vi "RomiSim_Write_Sensors.vi"(10 "Diff Drive Train Sim":T8 {"m_Motor"."Jr_KgM2" format="%13.5p"; "m_Motor"."L_H" format="%13.5p"; "m_Motor"."Kt_NMPerAmp" format="%13.5p"; "m_Motor"."KvINV_RadPerSecPerVolt" format="%13.5p"; "m_Motor"."R_Ohms" format="%13.5p"; "m_Motor"."FreeSpeed_RadPerSec" format="%13.5p"; "m_Motor"."FreeCurrent_Amps" format="%13.5p"; "m_Motor"."StallCurrent_Amps" format="%13.5p"; "m_Motor"."StallTorque_NM" format="%13.5p"; "m_Motor"."nominalVoltage_Volts" format="%13.5p"}, 11 "Counts/Feet":dbl) -> (0 "Right Speed Ft/Sec":dbl, 1 "Right Encoder":T6, 2 "Left Speed Ft/Sec":dbl, 3 "Left Encoder":T6, 4 "Robot Pose":T3 {"ROTATION"."SIN" format="%13.4f"; "ROTATION"."COS" format="%13.4f"; "ROTATION"."VALUE" format="%13.4f"; "TRANSLATION"."Y" format="%14.3f"; "TRANSLATION"."X" format="%14.3f"}, 5 "Gyro Deg":dbl, 7 "Gyro":T1)   [LabVIEW 2019]
uses:
  <vilib>/Rock Robotics/WPI/ThirdParty/JAS_Junk/TrajLib/TypeDef/DIFF_DRIVE_TRAIN_SIM.ctl
  <vilib>/Rock Robotics/WPI/ThirdParty/JAS_Junk/TrajLib/TypeDef/LINEAR_SYSTEM.ctl
  <vilib>/Analysis/Matrix/Datatypes/RealMatrix.ctl
  <vilib>/Rock Robotics/WPI/ThirdParty/JAS_Junk/TrajLib/TypeDef/DCMOTOR.CTL
  <vilib>/Rock Robotics/WPI/Simulation/Protocol/Devices/Encoder/Encoder proto.ctl
  <vilib>/Rock Robotics/WPI/Simulation/Protocol/Devices/Encoder/Encoder data protoo.ctl
  <vilib>/Rock Robotics/WPI/ThirdParty/JAS_Junk/TrajLib/TypeDef/POSE2D.ctl
  <vilib>/Rock Robotics/WPI/ThirdParty/JAS_Junk/TrajLib/TypeDef/TRANSLATION2D.ctl
  <vilib>/Rock Robotics/WPI/ThirdParty/JAS_Junk/TrajLib/TypeDef/ROTATION2D.ctl
  <vilib>/Rock Robotics/WPI/Simulation/Protocol/Devices/Gyro/Gyro proto.ctl
  <vilib>/Rock Robotics/WPI/Simulation/Protocol/Devices/Gyro/Gyro Data proto.ctl
  <vilib>/Rock Robotics/WPI/Simulation/Protocol/Devices/Encoder/Encoder Update Ops.ctl
  <vilib>/Rock Robotics/SystemInterfaces/Encoder/FPGA_EncoderIdx.ctl
  <vilib>/Rock Robotics/WPI/Simulation/Protocol/Devices/Gyro/Gyro Update Ops.ctl
  <vilib>/Rock Robotics/WPI/ThirdParty/JAS_Junk/TrajLib/Trajectory_Library.lvlib
  <vilib>/Rock Robotics/WPI/Simulation/Protocol/Devices/Encoder/Encoder Values.ctl
  <vilib>/Analysis/Matrix/NI_Matrix.lvlib
panel:
  # "<States, 1>"
  # "<Outputs, 1>"
  # "<Inputs, 1>"
  # "<Outputs, 1>"
  # "<States,States>"
  # "<States,Inputs>"
  # "<Outputs,States>"
  # "<Outputs,Inputs>"
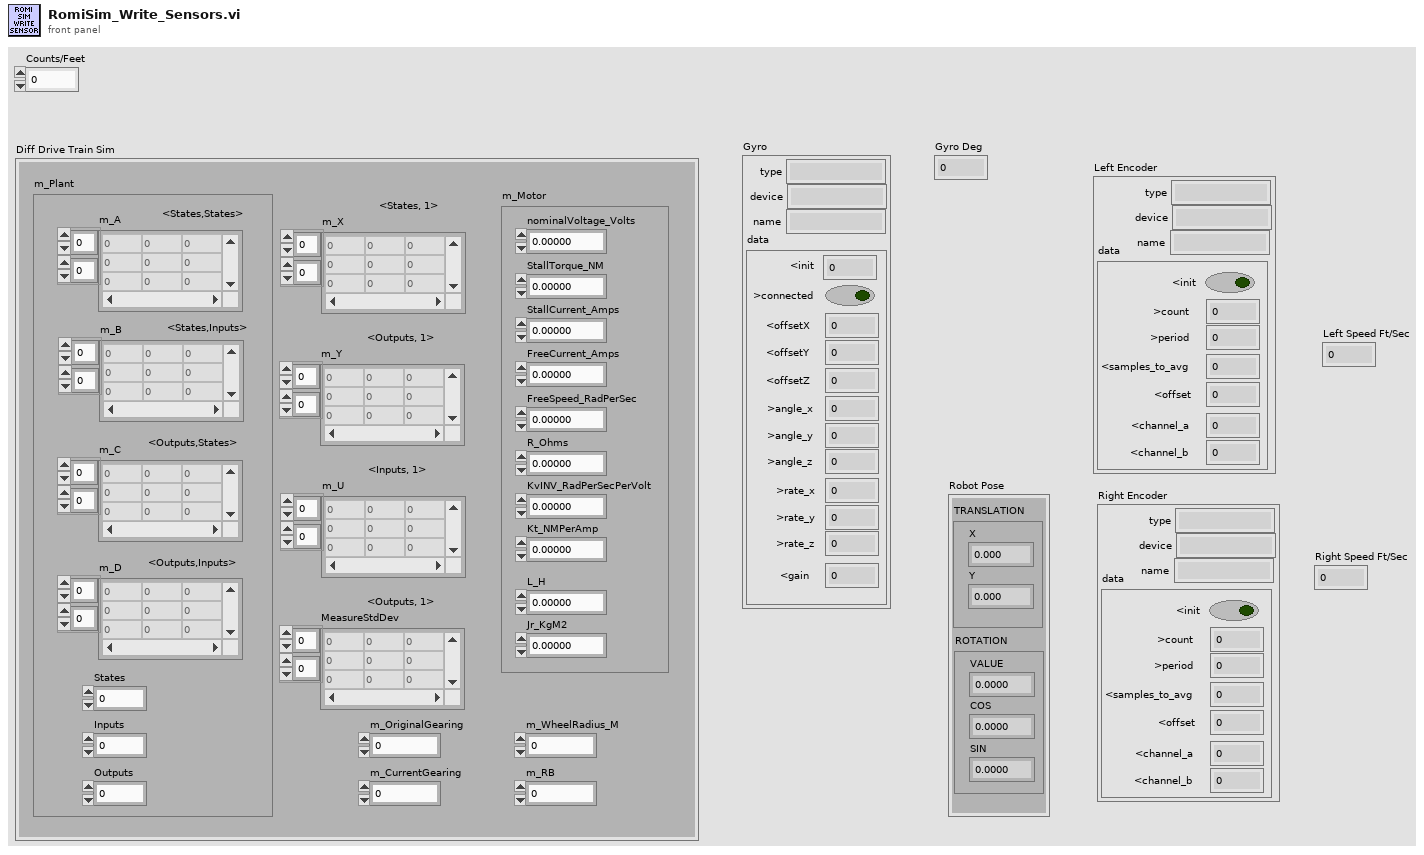
[diagram p1: front panel]
types:
  T1 = typedef "Gyro proto.ctl" = cluster{"type":string, "device":string, "name":string, "data":T2}
  T2 = typedef "Gyro Data proto.ctl" = cluster{"<init":i32, ">connected":bool, "<offsetX":dbl, "<offsetY":dbl, "<offsetZ":dbl, ">angle_x":dbl, ">angle_y":dbl, ">angle_z":dbl, ">rate_x":dbl, ">rate_y":dbl, ">rate_z":dbl, "<gain":dbl}
  T3 = typedef "Trajectory_Library.lvlib/POSE2D.ctl" = cluster{"TRANSLATION":T4, "ROTATION":T5}
  T4 = typedef "Trajectory_Library.lvlib/TRANSLATION2D.ctl" = cluster{"X":dbl, "Y":dbl}
  T5 = typedef "Trajectory_Library.lvlib/ROTATION2D.ctl" = cluster{"VALUE":dbl, "COS":dbl, "SIN":dbl}
  T6 = typedef "Encoder proto.ctl" = cluster{"type":string, "device":string, "name":string, "data":T7}
  T7 = typedef "Encoder data protoo.ctl" = cluster{"<init":bool, ">count":dbl, ">period":dbl, "<samples_to_avg":i32, "<offset":dbl, "<channel_a":i32, "<channel_b":i32}
  T8 = typedef "Trajectory_Library.lvlib/DIFF_DRIVE_TRAIN_SIM.ctl" = cluster{"m_Plant":T9, "m_X":T10, "m_Y":T10, "m_U":T10, "MeasureStdDev":T10, "m_Motor":T11, "m_OriginalGearing":dbl, "m_CurrentGearing":dbl, "m_WheelRadius_M":dbl, "m_RB":dbl}
  T9 = typedef "Trajectory_Library.lvlib/LINEAR_SYSTEM.ctl" = cluster{"m_A":T10, "m_B":T10, "m_C":T10, "m_D":T10, "States":i32, "Inputs":i32, "Outputs":i32}
  T10 = typedef "NI_Matrix.lvlib/RealMatrix.ctl" = dbl[][]
  T11 = typedef "Trajectory_Library.lvlib/DCMOTOR.CTL" = cluster{"nominalVoltage_Volts":dbl, "StallTorque_NM":dbl, "StallCurrent_Amps":dbl, "FreeCurrent_Amps":dbl, "FreeSpeed_RadPerSec":dbl, "R_Ohms":dbl, "KvINV_RadPerSecPerVolt":dbl, "Kt_NMPerAmp":dbl, "L_H":dbl, "Jr_KgM2":dbl}
  T12 = typedef "Encoder Values.ctl" = cluster{"Count":dbl, "Period":dbl}
  T13 = typedef "Gyro Update Ops.ctl" = enum16{"get", "delete", "JSON update", "set  name", "transmit initial", "reset", "set init", "set offsetX", "set offsetY", "set offsetZ", "set gain", "set angle X", "set angle Y", "set angle Z", "set rate X", "set rate Y", "set rate Z"}
  T14 = typedef "Encoder Update Ops.ctl" = enum16{"set init", "set count", "set period", "set reset", "set samples_to_avg", "get", "delete", "JSON update", "set name", "transmit initial", "reset", "set channel_a", "set channel_b", "set values"}
  T15 = typedef "FPGA_EncoderIdx.ctl" = enum8{"Enc 0", "Enc 1", "Enc 2", "Enc 3", "Enc 4", "Enc 5", "Enc 6", "Enc 7", "Invalid"}
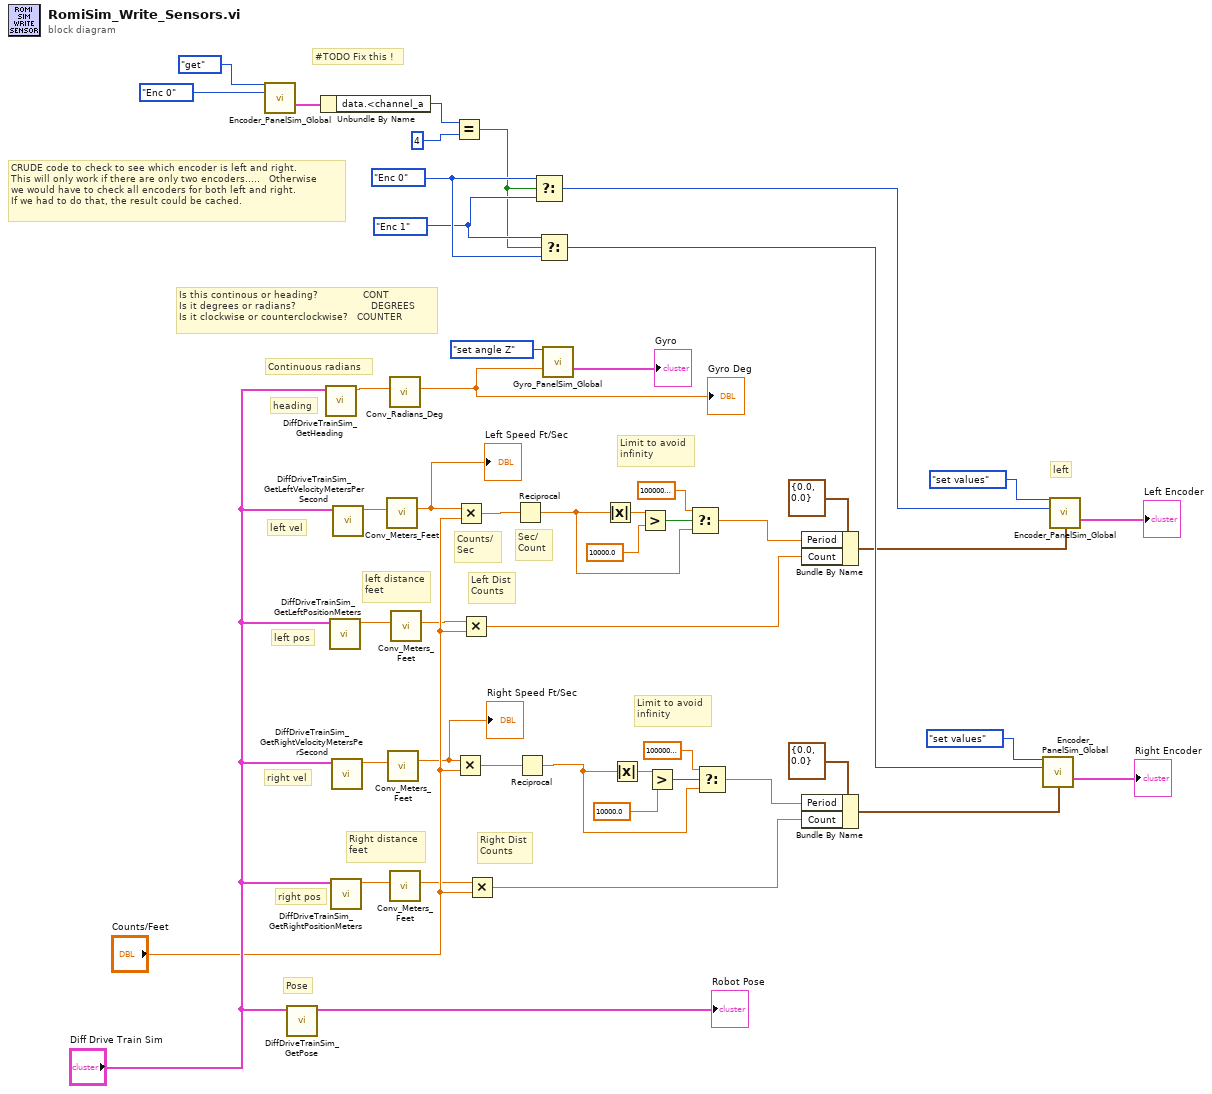
[diagram p0: block diagram]
diagram:
  w39 = FPGA_EncoderIdx."Enc 1" ("EncoderIndex")
  w40 = FPGA_EncoderIdx."Enc 0" ("EncoderIndex")
  # "#TODO Fix this !"
  # "Limit to avoid\ninfinity"
  # "left"
  # "CRUDE code to check to see which encoder is left and right.\nThis will only work if there are only two encoders.....   Otherwise\nwe would have to check all encoders for both left and right.\nIf we had to do that, the result could be cached."
  # "Right Dist\nCounts"
  # "Left Dist\nCounts"
  # "Is this continous or heading?               CONT\nIs it degrees or radians?                         DEGREES\nIs it clockwise or counterclockwise?   COUNTER"
  # "Sec/\nCount"
  # "Limit to avoid\ninfinity"
  # "Counts/\nSec"
  # "Continuous radians"
  # "Right distance\nfeet"
  # "left distance\nfeet"
  # "heading"
  # "left pos"
  # "right pos"
  # "right vel"
  # "left vel"
  # "Pose"
  n1 = call <vilib>:"Encoder_PanelSim_Global.vi"("menu"=Encoder_Update_Ops."get", "EncoderIndex"=FPGA_EncoderIdx."Enc 0") -> ("Encoder new"=w35:T6)  [unwired: 12 in, 1 out]
  n2 = call <vilib>:"DiffDriveTrainSim_GetPose.vi"("DiffDriveTrainSim"="Diff Drive Train Sim") -> ("Pose"=→"Robot Pose":T3)  [unwired: 10 in]
  n3 = Unbundle By Name(w35) -> ("data.<channel_a"=w36:i32)
  n4 = call <vilib>:"DiffDriveTrainSim_GetHeading.vi"("DiffDriveTrainSim"="Diff Drive Train Sim") -> ("Heading"=w46:dbl)  [unwired: 10 in]
  n5 = call <vilib>:"DiffDriveTrainSim_GetLeftPositionMeters.vi"("DiffDriveTrainSim"="Diff Drive Train Sim") -> ("LeftPosition_Meters"=w24:dbl)  [unwired: 10 in]
  n6 = call <vilib>:"DiffDriveTrainSim_GetRightPositionMeters.vi"("DiffDriveTrainSim"="Diff Drive Train Sim") -> ("RightPosition_Meters"=w21:dbl)  [unwired: 10 in]
  n7 = call <vilib>:"DiffDriveTrainSim_GetRightVelocityMetersPerSecond.vi"("DiffDriveTrainSim"="Diff Drive Train Sim") -> ("RightVel_M_Per_Sec"=w22:dbl)  [unwired: 10 in]
  n8 = call <vilib>:"DiffDriveTrainSim_GetLeftVelocityMetersPerSecond.vi"("DiffDriveTrainSim"="Diff Drive Train Sim") -> ("LeftVelocity_M_Per_Sec"=w23:dbl)  [unwired: 10 in]
  n9 = call <vilib>:"Conv_Meters_Feet.vi"("Meters"=w23) -> ("Feet"=w43:dbl)  [unwired: 10 in]
  "Left Speed Ft/Sec" <- w43
  n10 = call <vilib>:"Conv_Meters_Feet.vi"("Meters"=w22) -> ("Feet"=w25:dbl)  [unwired: 10 in]
  "Right Speed Ft/Sec" <- w25
  n11 = call <vilib>:"Conv_Radians_Deg.vi"("Radians"=w46) -> ("Degrees"=w47:dbl)  [unwired: 10 in]
  "Gyro Deg" <- w47
  n12 = call <vilib>:"Conv_Meters_Feet.vi"("Meters"=w21) -> ("Feet"=w30:dbl)  [unwired: 10 in]
  n13 = call <vilib>:"Conv_Meters_Feet.vi"("Meters"=w24) -> ("Feet"=w31:dbl)  [unwired: 10 in]
  n14 = Equal?(x=w36, y=4) -> (x = y?=w38:bool)
  n15 = Multiply(x=w25, y="Counts/Feet") -> (x*y=w26:dbl)
  n16 = Multiply(x=w43, y="Counts/Feet") -> (x*y=w27:dbl)
  n17 = Multiply(x=w31, y="Counts/Feet") -> (x*y=w5:dbl)
  n18 = Multiply(x=w30, y="Counts/Feet") -> (x*y=w9:dbl)
  n19 = Reciprocal(x=w27) -> (1/x=w29:dbl)
  n20 = Reciprocal(x=w26) -> (1/x=w28:dbl)
  n21 = Select(t=w40, s=w38, f=w39) -> (s? t:f=w41:T15)
  n22 = Select(t=w39, s=w38, f=w40) -> (s? t:f=w42:T15)
  n23 = call <vilib>:"Gyro_PanelSim_Global.vi"("Menu"=Gyro_Update_Ops."set angle Z", "Numeric Value"=w47) -> ("Value out"=→"Gyro":T1)  [unwired: 12 in, 1 out]
  n24 = Absolute Value(x=w29) -> (abs(x)=w12:dbl)
  n25 = Absolute Value(x=w28) -> (abs(x)=w16:dbl)
  n26 = Greater?(x=w12, y=10000.0) -> (0:w14:bool)
  n27 = Greater?(x=w16, y=10000.0) -> (0:w18:bool)
  n28 = Select(t=100000000000000.0, s=w14, f=w29) -> (s? t:f=w6:dbl)
  n29 = Select(t=100000000000000.0, s=w18, f=w28) -> (s? t:f=w8:dbl)
  n30 = Bundle By Name(cluster=T12 {"Count"=0.0, "Period"=0.0} ("Encoder Values"), "Period"=w6, "Count"=w5) -> (w4:T12)
  n31 = Bundle By Name(cluster=T12 {"Count"=0.0, "Period"=0.0} ("Encoder Values"), "Period"=w8, "Count"=w9) -> (w2:T12)
  n32 = call <vilib>:"Encoder_PanelSim_Global.vi"("menu"=Encoder_Update_Ops."set values", "EncoderIndex"=w42, "Values"=w2) -> ("Encoder new"=→"Right Encoder":T6)  [unwired: 11 in, 1 out]
  n33 = call <vilib>:"Encoder_PanelSim_Global.vi"("menu"=Encoder_Update_Ops."set values", "EncoderIndex"=w41, "Values"=w4) -> ("Encoder new"=→"Left Encoder":T6)  [unwired: 11 in, 1 out]
